vi "Configure Output Angle.vi"(0 "VISA resource name":refnum<visa-resource-name>, 5 "Start Angle (0)":i32 min=0 max=359, 7 "End Angle: (0)":i32 min=0 max=359, 11 "error in (no error)":errorcluster) -> (4 "VISA resource name out":refnum<visa-resource-name>, 15 "error out":errorcluster)   [LabVIEW 2016, in "APT 300XAC Series.lvlib"]
doc: "Configures the <B>start angle and end angle of the sine wave output</B> in the power source instrument.\n\nNote :\nThe Output Angle parameter type is a step parameter.\n\nAssociated Power Technologies feature that provides the flexibility to monitor current conditions under different starting / ending angles of the sine wave.\nThe actual degree angle from 0 - 359 in which the AC waveform output will begin."
uses:
  APT 300XAC Series.lvlib
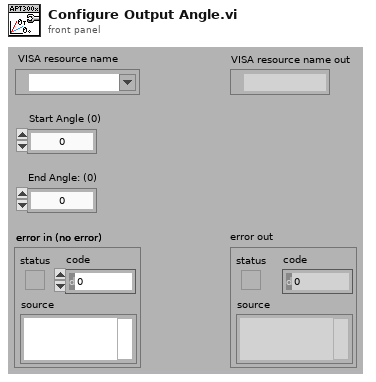
[diagram p1: front panel]
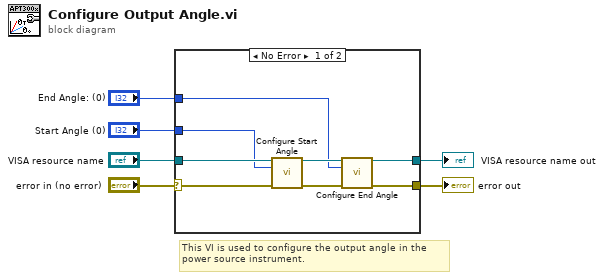
[diagram p0: block diagram]
diagram:
  # "This VI is used to configure the output angle in the\npower source instrument."
  n1 = case shown="No Error" "error in (no error)" {
    selector: "error in (no error)" -> [w9 w15]
    tunnel: "VISA resource name" -> [w14 w16]
    tunnel: [w13 w16] -> w5
    tunnel: [w12 w15] -> w4
    tunnel: "End Angle: (0)" -> [w8 _]
    tunnel: "Start Angle (0)" -> [w7 _]
    frame No Error {
      n2 = call "Configure Start Angle.vi"("VISA resource name"=w14, "Start Angle (0)"=w7, "error in (no error)"=w9) -> ("VISA resource name out"=w11:refnum<visa-resource-name>, "error out"=w10:errorcluster)  [unwired: 11 in]
      n3 = call "Configure End Angle.vi"("VISA resource name"=w11, "End Angle: (0)"=w8, "error in (no error)"=w10) -> ("VISA resource name out"=w13:refnum<visa-resource-name>, "error out"=w12:errorcluster)  [unwired: 11 in]
    }
    frame Error {
    }
  }
  "error out" <- w4
  "VISA resource name out" <- w5
